vi "Get Data.vi"(8 "error in (no error)":errorcluster, 10 "Bus In":refnum<class "Bus.lvclass">, 11 "Query in":refnum<class "Query.lvclass">) -> (0 "error out":errorcluster, 1 "String Read":string, 2 "Bus Out":refnum<class "Bus.lvclass">, 3 "Query out":refnum<class "Query.lvclass">)   [LabVIEW 2018, in "Query.lvclass"]
doc: "Query.lvclass:Get Data.vi\n\nThis is the template for the Get Data VI for the Query class.\n\nInstrument Communication Module Version 1.0\nSeptember, 2017 Original Code Consulting David Thomson\n www.originalcode.com"
uses:
  Query.lvclass
  Bus/Bus.lvclass
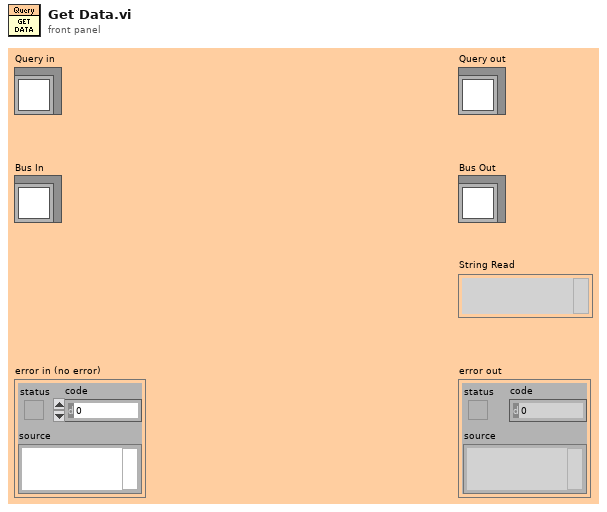
[diagram p1: front panel]
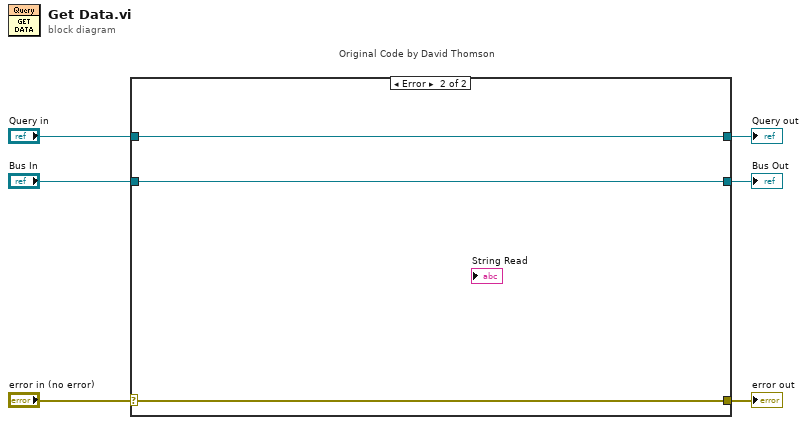
[diagram p0: block diagram]
diagram:
  n1 = case "Original Code by David Thomson" shown="Error" "error in (no error)" {
    selector: "error in (no error)" -> [w8 w12]
    tunnel: [w8 w12] -> w5
    tunnel: [w9 w11] -> w3
    tunnel: "Query in" -> [w9 w11]
    tunnel: [w7 w10] -> w2
    tunnel: "Bus In" -> [w7 w10]
    frame No Error {
    }
    frame Error {
    }
  }
  "error out" <- w5
  "Query out" <- w3
  "Bus Out" <- w2
